vi "Get Account Information.vi"(6 "Account Number":string, 8 "error in (no error)":errorcluster, 11 "Bank Account in":refnum<class "Bank Account.lvclass">) -> (0 "error out":errorcluster, 3 "Bank Account out":refnum<class "Bank Account.lvclass">, 4 "Account Verified?":bool)   [LabVIEW 2016, in "CLD Exam - ATM.lvlib" / "Bank Account.lvclass"]
uses:
  Bank Account.lvclass
  Bank Account.lvclass/Bank Account.ctl
  <vilib>/Utility/file.llb/Read Delimited Spreadsheet (string).vi
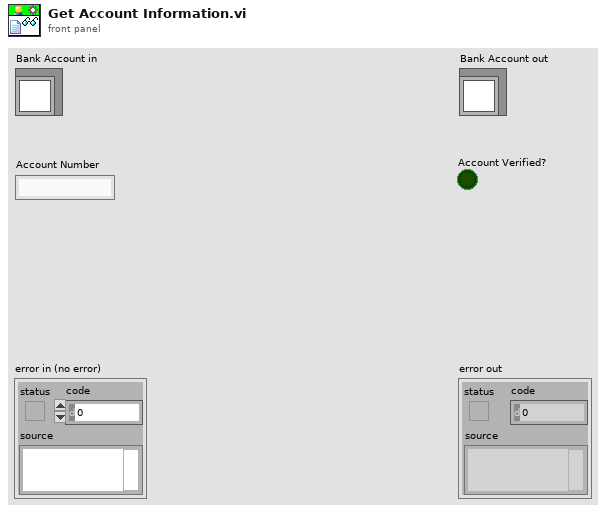
[diagram p1: front panel]
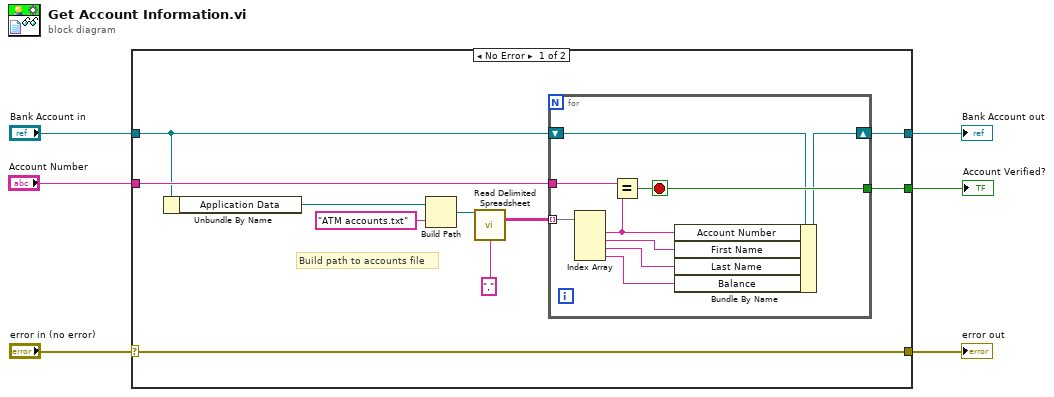
[diagram p0: block diagram]
diagram:
  n1 = case shown="No Error" "error in (no error)" {
    selector: "error in (no error)" -> [w16 w27]
    tunnel: [w16 w27] -> w5
    tunnel: [w7 w26] -> w3
    tunnel: "Bank Account in" -> [w8 w26]
    tunnel: "Account Number" -> [w10 _]
    tunnel: [w9 _] -> w1
    frame No Error {
      # "Build path to accounts file"
      n2 = Unbundle By Name(w8) -> ("Application Data"=w14:path)
      n3 = Build Path(base path=w14, name or relative path="ATM accounts.txt") -> (appended path=w13:path)
      n4 = call-poly <vilib>:"Read Delimited Spreadsheet.vi"("file path (dialog if empty)"=w13, "delimiter (\\t)"="," ("delimiter (\\t)")) -> ("all rows"=w11:string[][])  [unwired: 8 in, 5 out]
      n5 = for {
        tunnel: w11 -> [w25] mode=indexing
        tunnel: w10 -> [w24]
        tunnel: [w23] -> w9
        shift-right: [w17] -> w7
        shift-left: w8 -> [w18]
        stop <- w23 stop-if-true
        n6 = Index Array(array=w25) -> (element #1=w22:string, element #2=w21:string, element #3=w20:string, element #4=w19:string)  [unwired: 4 in]
        n7 = Equal?(x=w24, y=w22) -> (x = y?=w23:bool)
        n8 = Bundle By Name(cluster=w18, "Account Number"=w22, "First Name"=w21, "Last Name"=w20, "Balance"=w19) -> (w17:refnum<class "Bank Account.lvclass">)
      }
    }
    frame Error {
    }
  }
  "error out" <- w5
  "Bank Account out" <- w3
  "Account Verified?" <- w1
